vi "Read Power Monitor Data.vi"(8 "error in (no error)":errorcluster, 10 "Data File Path":path, 11 "BFECC in":refnum<class "BFECC.lvclass">) -> (0 "error out":errorcluster, 2 "Data":T1, 3 "BFECC out":refnum<class "BFECC.lvclass">)   [LabVIEW 2018, in "BFECC.lvlib" / "BFECC.lvclass"]
uses:
  BFECC.lvclass
  Custom Controls/Supply List.ctl
  <vilib>/addons/_JKI.lib/Serialization/JSON/JKI JSON Serialization.lvlib
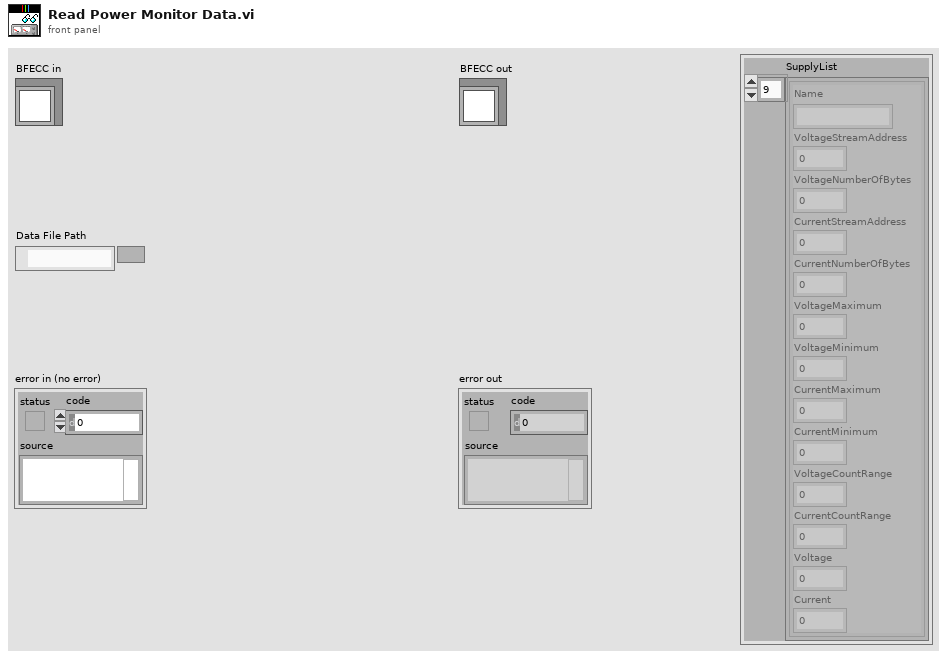
[diagram p1: front panel]
types:
  T1 = typedef "BFECC.lvlib/BFECC.lvclass/Supply List.ctl" = cluster{"SupplyList":cluster{"Name":string, "VoltageStreamAddress":i32, "VoltageNumberOfBytes":i32, "CurrentStreamAddress":i32, "CurrentNumberOfBytes":i32, "VoltageMaximum":dbl, "VoltageMinimum":dbl, "CurrentMaximum":dbl, "CurrentMinimum":dbl, "VoltageCountRange":i32, "CurrentCountRange":i32, "Voltage":dbl, "Current":dbl}[]}
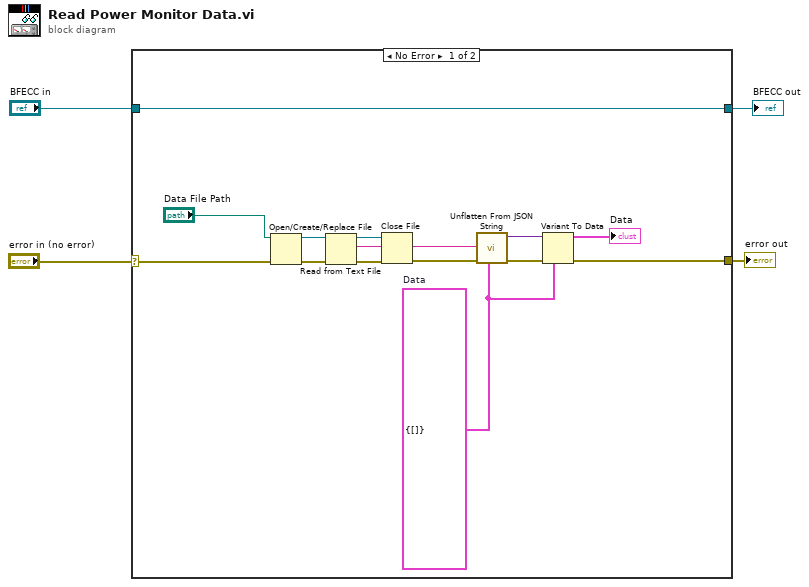
[diagram p0: block diagram]
diagram:
  n1 = case shown="No Error" "error in (no error)" {
    selector: "error in (no error)" -> [w16 w20]
    tunnel: [w7 w20] -> w3
    tunnel: [w18 w19] -> w1
    tunnel: "BFECC in" -> [w18 w19]
    frame No Error {
      w6 = T1 {"SupplyList"=[]}  # Data
      n2 = Open/Create/Replace File(file path (use dialog)="Data File Path", error in=w16) -> (refnum out=w14:refnum<file>, error out=w15:errorcluster)  [unwired: 4 in, 1 out]
      n3 = Read from Text File(file (use dialog)=w14, error in=w15) -> (refnum out=w12:refnum<file>, text=w11:string, error out=w13:errorcluster)  [unwired: 2 in, 1 out]
      n4 = Close File(refnum=w12, error in=w13) -> (error out=w9:errorcluster)  [unwired: 1 out]
      n5 = call <vilib>:"Unflatten From JSON String.vi"("Type and Defaults"=w6, "error in (no error)"=w9, "JSON String"=w11) -> ("error out"=w8:errorcluster, "Variant"=w10:variant)  [unwired: 7 in]
      n6 = Variant To Data(error in=w8, type=w6, Variant=w10) -> (data=→"Data":T1, error out=w7:errorcluster)
    }
    frame Error {
    }
  }
  "error out" <- w3
  "BFECC out" <- w1
